vi "ClassPanel.vi"(8 "error in (no error)":errorcluster caption="entrée d'erreur (pas d'erreur)", 11 "DefaultDev.lvclass":refnum<class "DefaultDev.lvclass">) -> (0 "error out":errorcluster caption="sortie d'erreur", 3 "DefaultDev.lvclass Out":refnum<class "DefaultDev.lvclass">)   [LabVIEW 2019, in "DefaultDev.lvclass"]
uses:
  DefaultDev.lvclass
  C:/Programmes Labview/LabscanV1A/DevicesClass/BaseDevice/BaseDevice.lvclass
  DevicesClass/BaseDevice/Accessor/GetClassEvent.vi
panel:
  out "ControlsNames":string[](array[string])
  in  "Con/Disc.":bool
  in  "MainProgQ":refnum<queue>
  in  "MainProgQEvent":refnum<user-event>
  in  "Acq":bool
  in  "Stop":bool
  out "2":dbl format="%<%H:%M:%S%1u>t"
  in  "MiseAJour":bool
  in  "1":dbl=60.0 min=0.1 step=0.1 format="%#.1f"
  out "Init Program":bool
  # "DefaultDevice"
  # "this MUST labeled with class name"
  # "this MUST be present and labeled \"Stop\" and \"Acq\""
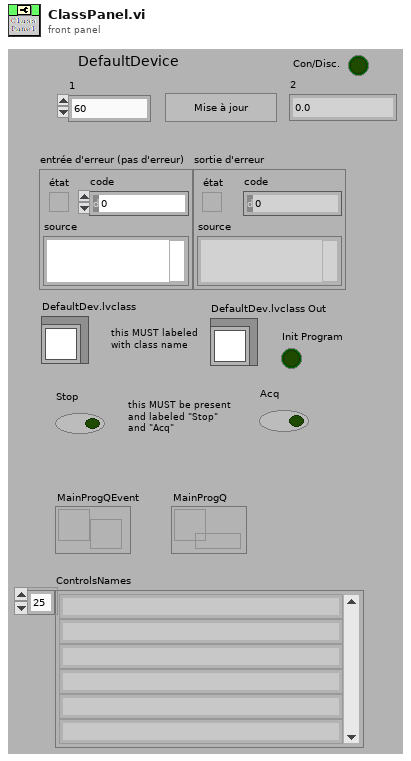
[diagram p1: front panel]
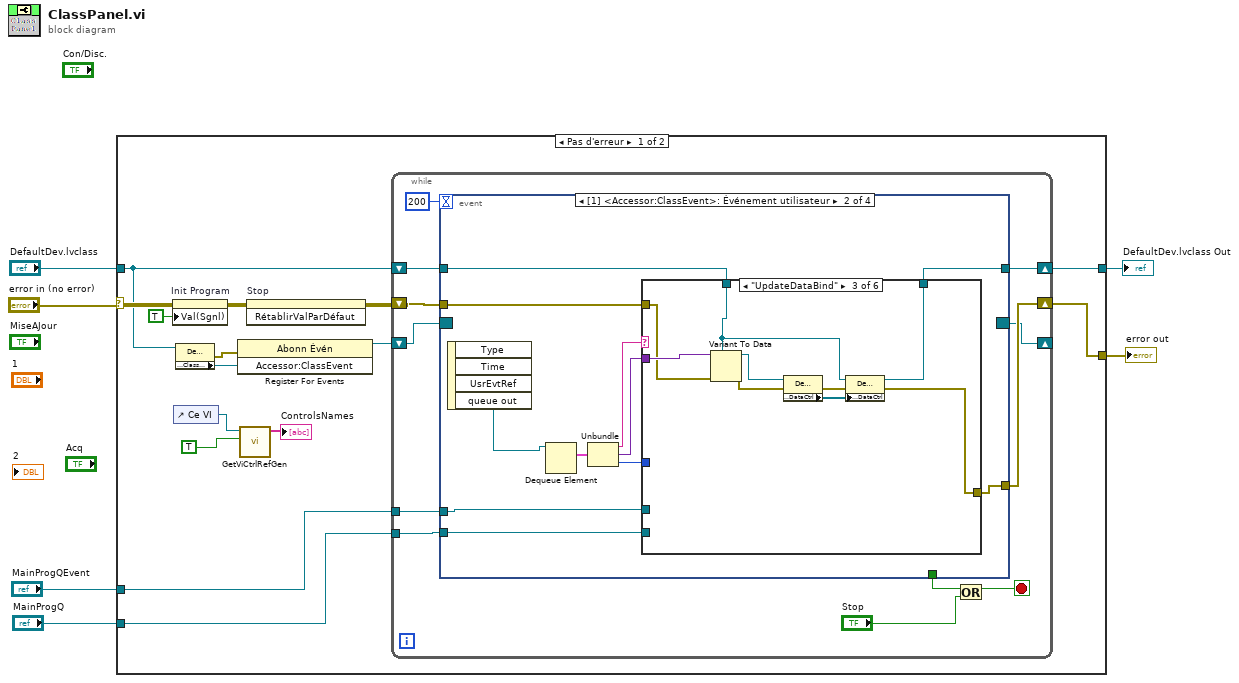
[diagram p0: block diagram]
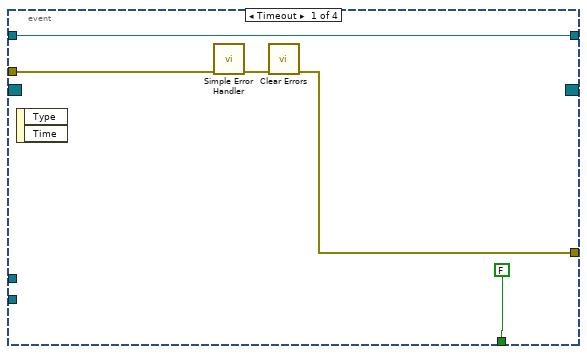
[diagram p2: hidden frame]
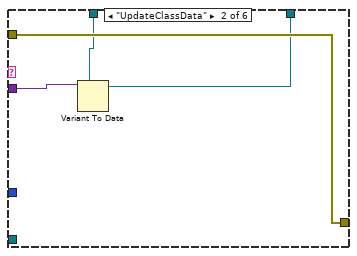
[diagram p4: hidden frame]
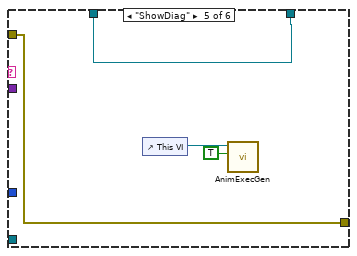
[diagram p6: hidden frame]
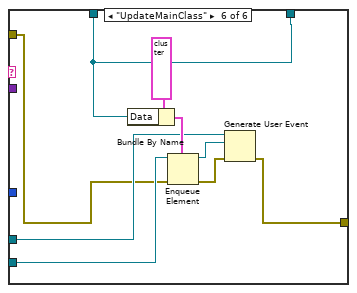
[diagram p7: hidden frame]
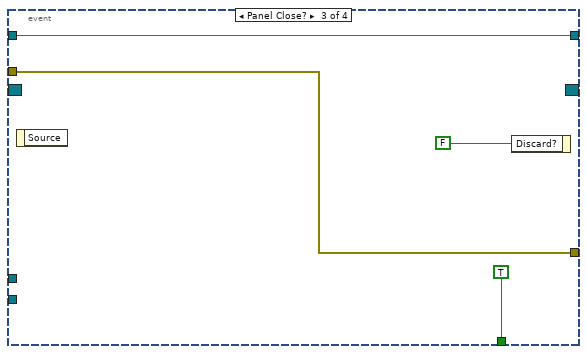
[diagram p8: hidden frame]
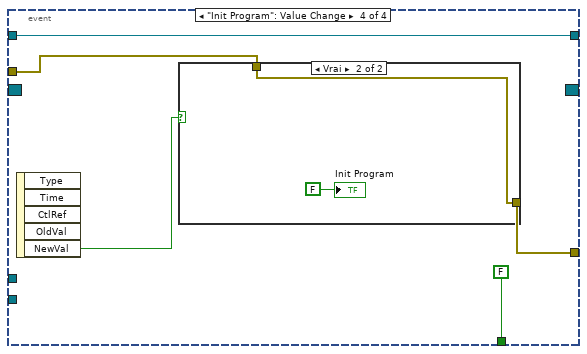
[diagram p9: hidden frame]
diagram:
  n1 = case shown="Pas d'erreur" "error in (no error)" {
    selector: "error in (no error)" -> [w18 w93]
    tunnel: [w21 w93] -> w5
    tunnel: "DefaultDev.lvclass" -> [w13 w92]
    tunnel: [w19 w92] -> w3
    tunnel: "MainProgQEvent" -> [w11 _]
    tunnel: "MainProgQ" -> [w10 _]
    frame No Error {
      n2 = property on="Init Program" class="Bool (strict)"(error in=w18, "Val(Sgnl)"=TRUE ("Valeur (Signalisation)")) -> (error out=w17:errorcluster)  [unwired: 1 in, 1 out]
      n3 = control-ref of="Ce VI"() -> (w8:refnum<vi>)
      n4 = property class="DefaultDev.lvclass"(reference=w13) -> (error out=w15:errorcluster, "Accessor:ClassEvent"=w14:refnum<user-event>)  [unwired: 1 in, 1 out]
      n5 = register-events(error in=w15, w14) -> (reference out=w12:refnum<event-registration>)  [unwired: 1 in, 1 out]
      n6 = call <userlib>:"GetViCtrlRefGen.vi"("InclTabCTrl"=TRUE, "VIRef"=w8) -> ("ControlsNames"=→"ControlsNames":string[])  [unwired: 7 in, 2 out]
      n7 = invoke on="Stop" class="Bool (strict)" method="RétablirValParDéfaut"(error in=w17) -> (error out=w16:errorcluster)  [unwired: 2 in, 2 out]
      n8 = while {
        shift-right: [w31] -> w21
        shift-left: w16 -> [w32]
        shift-right: [w28] -> w19
        shift-left: w13 -> [w30]
        shift-right: [w24] -> _
        shift-left: w12 -> [w25]
        tunnel: w11 -> [w23]
        tunnel: w10 -> [w22]
        stop <- w27 stop-if-true
        n9 = event shown="[1] <Accessor:ClassEvent>: Événement utilisateur" {
          selector: w25 -> [_ _ _ _]
          dyn-events: [_ _ _ _] -> w24
          timeout: 200 -> [_ _ _ _]
          tunnel: w32 -> [w36 w48 w81 w87]
          tunnel: [w34 w42 w81 w86] -> w31
          tunnel: w30 -> [w37 w49 w80 w85]
          tunnel: [FALSE _ TRUE FALSE] -> w29
          tunnel: [w37 w41 w80 w85] -> w28
          tunnel: w23 -> [_ w40 _ _]
          tunnel: w22 -> [_ w39 _ _]
          event Timeout {
            n10 = event-data() -> ()  [unwired: 1 in, 2 out]
            n11 = call <vilib>:"Simple Error Handler.vi"("error in (no error)"=w36) -> ("error out"=w35:errorcluster)  [unwired: 4 in, 4 out]
            n12 = call <vilib>:"Clear Errors.vi"("error in (no error)"=w35) -> ("error out"=w34:errorcluster)  [unwired: 5 in, 1 out]
          }
          event User Event {
            n13 = event-data() -> ("queue out"=w46:refnum<queue>)  [unwired: 1 in, 3 out]
            n14 = Dequeue Element(queue=w46) -> (element=w47:cluster{"Message":string, "Data":variant, i32})  [unwired: 2 in, 3 out]
            n15 = Unbundle(w47) -> ("Message"=w45:string, "Data"=w44:variant, w43:i32)
            n16 = case shown="\"UpdateDataBind\"" w45 {
              tunnel: w48 -> [w51 w55 w59 w65 w69 w72]
              tunnel: w44 -> [_ w54 w64 _ _ _]
              tunnel: w49 -> [w50 w53 w56 w66 w70 w75]
              tunnel: [w50 w52 w57 w66 w70 w75] -> w41
              tunnel: [w51 w55 w58 w65 w69 w71] -> w42
              tunnel: w43 -> [_ _ _ _ _ _]
              tunnel: w40 -> [_ _ _ _ _ w74]
              tunnel: w39 -> [_ _ _ _ _ w73]
              frame Default {
              }
              frame "UpdateClassData" {
                n17 = Variant To Data(type=w53, Variant=w54) -> (data=w52:refnum<class "DefaultDev.lvclass">)  [unwired: 1 in, 1 out]
              }
              frame "UpdateDataBind" {
                n18 = Variant To Data(error in=w59, type=w56, Variant=w64) -> (data=w61:refnum<class "DefaultDev.lvclass">, error out=w60:errorcluster)
                n19 = property class="DefaultDev.lvclass"(reference=w61, error in=w60) -> (error out=w63:errorcluster, "Accessor:DataCtrl"=w62:refnum<vi>[])  [unwired: 1 out]
                n20 = property class="DefaultDev.lvclass"(reference=w56, error in=w63, "Accessor:DataCtrl"=w62) -> (reference out=w57:refnum<class "DefaultDev.lvclass">, error out=w58:errorcluster)
              }
              frame "MeasDone" {
              }
              frame "ShowDiag" {
                n21 = control-ref of="This VI"() -> (w68:refnum<vi>)
                n22 = call <userlib>:"AnimExecGen.vi"("Animer l'exécution ?"=TRUE, "ViRef"=w68) -> ()  [unwired: 9 in, 1 out]
              }
              frame "UpdateMainClass" {
                n23 = Bundle By Name(cluster=cluster{"Message":string, "Data":variant, i32} {"Message"="", "Data"=variant, 0} ("élément"), "Data"=w75) -> (w76:cluster{"Message":string, "Data":variant, i32})
                n24 = Enqueue Element(queue=w73, element=w76, error in (no error)=w72) -> (queue out=w79:refnum<queue>, error out=w78:errorcluster)  [unwired: 1 in, 1 out]
                n25 = Generate User Event(user event=w74, event data cluster=w79, error in=w78) -> (error out=w71:errorcluster)  [unwired: 1 in, 1 out]
              }
            }
          }
          event Panel Close? {
            n26 = event-data() -> ()  [unwired: 1 in, 1 out]
            n27 = event-data("Discard?"=FALSE ("Rejeter ?")) -> ()  [unwired: 1 in, 1 out]
          }
          event "Init Program": Value Change {
            n28 = event-data() -> ("NewVal"=w88:bool)  [unwired: 1 in, 4 out]
            n29 = case shown="Vrai" w88 {
              tunnel: w87 -> [w89 w90]
              tunnel: [w89 w90] -> w86
              frame False {
              }
              frame True {
                "Init Program" <- FALSE
              }
            }
          }
        }
        n30 = Or(x=w29, y="Stop") -> (x .or. y?=w27:bool)
      }
    }
    frame Error {
    }
  }
  "error out" <- w5
  "DefaultDev.lvclass Out" <- w3
